vi "Sub_PLC_AllBitDisplay.vi"(11 "入力":u8[](array[numeric])) -> (2 "AllByte_Array":bool[][](array[boolean]), 3 "AllByte_Cluster":cluster{"1byte":bool[]}[](array[cluster]))   [LabVIEW 2018]
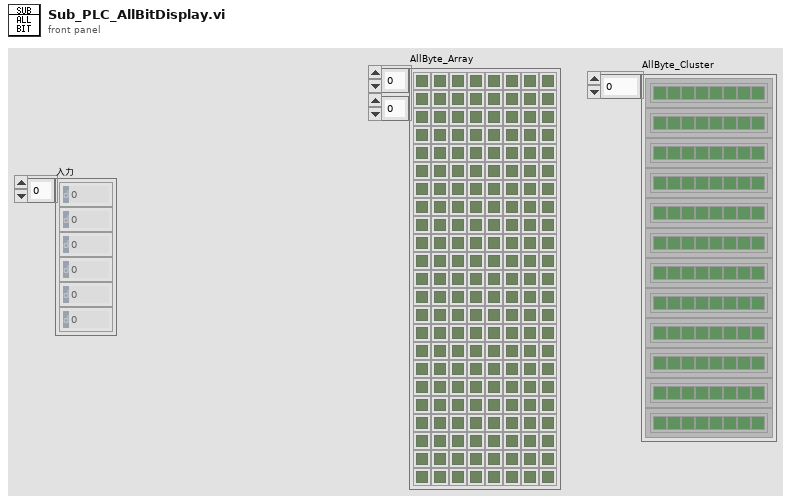
[diagram p1: front panel]
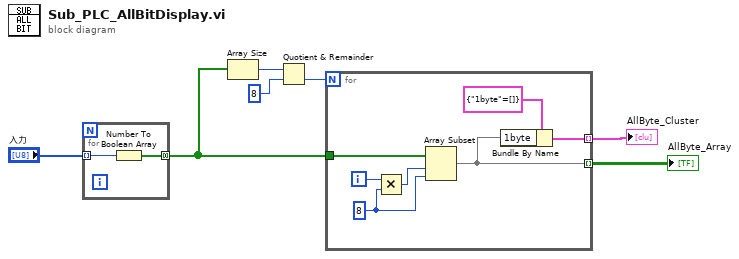
[diagram p0: block diagram]
diagram:
  n1 = for {
    tunnel: "入力" -> [w9] mode=indexing
    tunnel: [w8] -> w3 mode=concatenating
    n2 = Number To Boolean Array(number=w9) -> (Boolean array=w8:bool[])
  }
  n3 = Array Size(array=w3) -> (size(s)=w7:i32)
  n4 = Quotient & Remainder(x=w7, y=8) -> (floor(x/y)=w1:i32)  [unwired: 1 out]
  n5 = for {
    N: w1 -> [_]
    tunnel: w3 -> [w16]
    tunnel: [w11] -> w5 mode=indexing
    tunnel: [w10] -> w2 mode=indexing
    i -> [w15]
    w13 = 8
    n6 = Multiply(x=w15, y=w13) -> (x*y=w14:i32)
    n7 = Array Subset(array=w16, index=w14, length=w13) -> (w11:bool[])
    n8 = Bundle By Name(cluster=cluster{"1byte":bool[]} {"1byte"=[]} ("クラスタ"), "1byte"=w11) -> (w10:cluster{"1byte":bool[]})
  }
  "AllByte_Array" <- w5
  "AllByte_Cluster" <- w2
